vi "Conifg Dump.vi"(8 "error in (no error)":errorcluster, 11 "Sections":T1(array[cluster])) -> (0 "error out":errorcluster, 3 "Text":string)   [LabVIEW 2018]
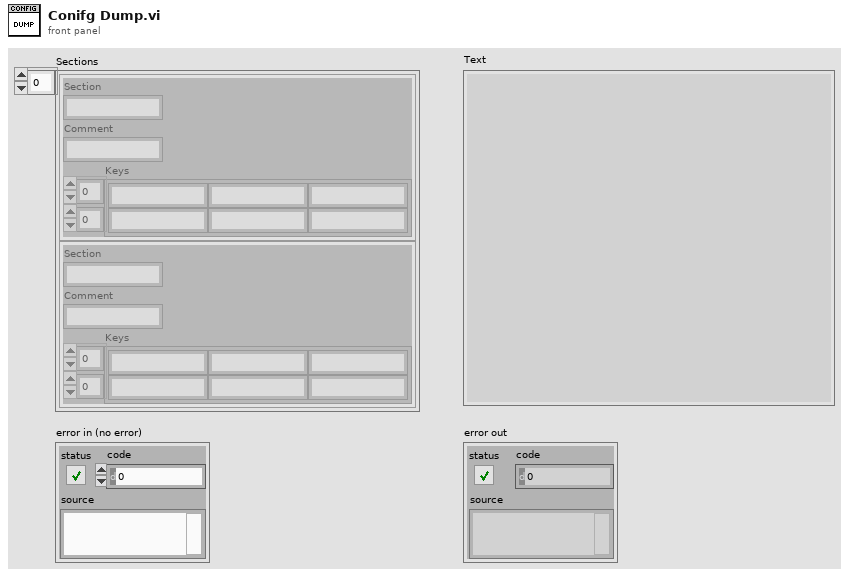
[diagram p1: front panel]
types:
  T1 = cluster{"Section":string, "Comment":string, "Keys":string[][]}[]
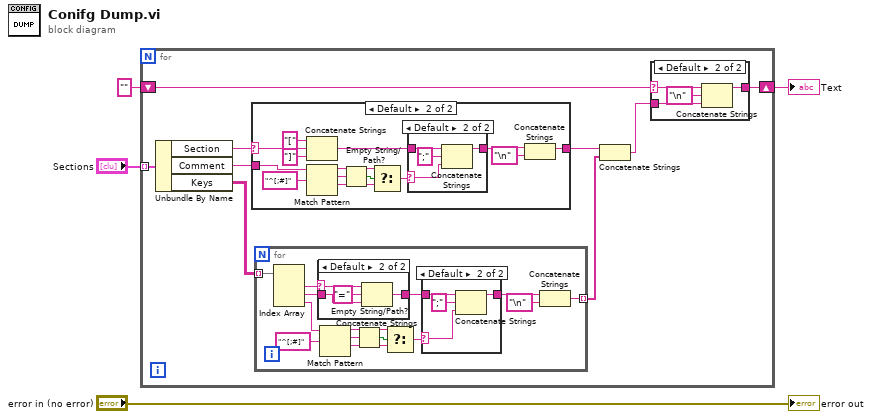
[diagram p0: block diagram]
diagram:
  n1 = for {
    tunnel: "Sections" -> [w13] mode=indexing
    shift-right: [w6] -> w1
    shift-left: "" -> [w5]
    n2 = Unbundle By Name(w13) -> ("Section"=w12:string, "Comment"=w11:string, "Keys"=w10:string[][])
    n3 = case shown="Default" w12 {
      selector: w12 -> [_ w55]
      tunnel: w11 -> [_ w45]
      tunnel: [_ w42] -> w8
      frame "" {
      }
      frame Default {
        n4 = Concatenate Strings("[" ("string"), w55, "]" ("string")) -> (w46:string)
        n5 = Match Pattern(string=w45, regular expression="^[;#]") -> (before substring=w51:string, match substring=w49:string, after substring=w50:string)  [unwired: 1 in, 1 out]
        n6 = Empty String/Path?(string/path=w49) -> (empty?=w48:bool)
        n7 = Select(t=w51, s=w48, f=w50) -> (s? t:f=w47:string)
        n8 = case shown="Default" w47 {
          selector: w47 -> [_ w59]
          tunnel: w46 -> [w56 w58]
          tunnel: [w56 w57] -> w43
          frame "" {
          }
          frame Default {
            n9 = Concatenate Strings(w58, ";" ("string"), w59) -> (w57:string)
          }
        }
        n10 = Concatenate Strings(w43, "\n" ("string")) -> (w42:string)
      }
    }
    n11 = for {
      tunnel: w10 -> [w32] mode=indexing
      tunnel: [w19] -> w9 mode=indexing
      n12 = Index Array(array=w32) -> (element #1=w25:string, element #2=w24:string, element #3=w22:string)  [unwired: 3 in]
      n13 = case shown="Default" w25 {
        selector: w25 -> [_ w36]
        tunnel: w24 -> [_ w34]
        tunnel: [_ w33] -> w23
        frame "" {
        }
        frame Default {
          n14 = Concatenate Strings(w36, "=" ("string"), w34) -> (w33:string)
        }
      }
      n15 = Match Pattern(string=w22, regular expression="^[;#]") -> (before substring=w27:string, match substring=w29:string, after substring=w28:string)  [unwired: 1 in, 1 out]
      n16 = Empty String/Path?(string/path=w29) -> (empty?=w30:bool)
      n17 = Select(t=w27, s=w30, f=w28) -> (s? t:f=w31:string)
      n18 = case shown="Default" w31 {
        selector: w31 -> [_ w40]
        tunnel: w23 -> [w37 w39]
        tunnel: [w37 w38] -> w21
        frame "" {
        }
        frame Default {
          n19 = Concatenate Strings(w39, ";" ("string"), w40) -> (w38:string)
        }
      }
      n20 = Concatenate Strings(w21, "\n" ("string")) -> (w19:string)
    }
    n21 = Concatenate Strings(w8, w9) -> (w7:string)
    n22 = case shown="Default" w5 {
      selector: w5 -> [_ w17]
      tunnel: [w14 w18] -> w6
      tunnel: w7 -> [w14 w15]
      frame "" {
      }
      frame Default {
        n23 = Concatenate Strings(w17, "\n" ("string"), w15) -> (w18:string)
      }
    }
  }
  "Text" <- w1
  "error out" <- "error in (no error)"
